vi "ConvertInsightPropertyToTdmsProperty_i32.vi"(9 "Tdms Property Name":string, 10 "Insight Property Name":string, 11 "Insight Properties":T2[](array[typedef])) -> (3 "Tdms Properties":T1[](array[typedef]))   [LabVIEW 2017, in "Tdms.lvlib"]
uses:
  <vilib>/addons/InsightCM/Utilities/Tdms/Tdms.lvlib
  <vilib>/addons/InsightCM/MessageBus/Base/controls/KeyValuePair.ctl
  <vilib>/addons/InsightCM/Utilities/Tdms/controls/Property.ctl
  <vilib>/addons/InsightCM/Utilities/PropertyHelpers/PropertyHelpers.lvlib
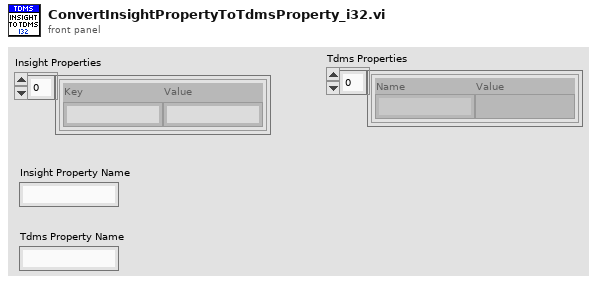
[diagram p1: front panel]
types:
  T1 = typedef "Tdms.lvlib/Property.ctl" = cluster{"Name":string, "Value":variant}
  T2 = typedef "KeyValuePair.ctl" = cluster{"Key":string, "Value":string}
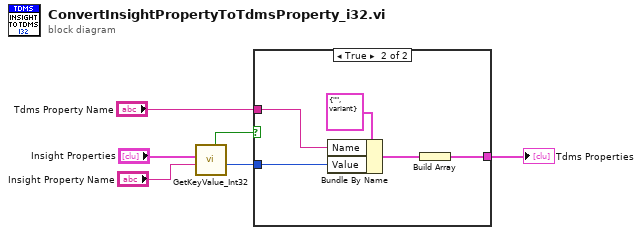
[diagram p0: block diagram]
diagram:
  n1 = call <vilib>:"GetKeyValue_Int32.vi"("key"="Insight Property Name", "key value pairs"="Insight Properties") -> ("value"=w3:i32, "found"=w4:bool)  [unwired: 7 in, 1 out]
  n2 = case shown="True" w4 {
    tunnel: "Tdms Property Name" -> [_ w11]
    tunnel: w3 -> [_ w10]
    tunnel: [_ w7] -> w5
    frame False {
    }
    frame True {
      n3 = Bundle By Name(cluster=T1 {"Name"="", "Value"=variant} ("Property"), "Name"=w11, "Value"=w10) -> (w8:T1)
      n4 = Build Array(w8) -> (w7:T1[])
    }
  }
  "Tdms Properties" <- w5
